vi "Handle.vi"(10 "log record":T1 {"timestamp" format="%<%x %.3X>T"}, 11 "string handler in":refnum<class "String Handler.lvclass">) -> (0 "writer error":errorcluster, 1 "formatter error":errorcluster, 3 "string handler out":refnum<class "String Handler.lvclass">)   [LabVIEW 2024, in "Logging.lvlib" / "String Handler.lvclass"]
uses:
  String Handler.lvclass
  String Handler.lvclass/String Handler.ctl
  Formatters/Formatter/Formatter.lvclass
  Log Record.ctl
  Logging.lvlib
  Logger/Internal Log Levels.ctl
panel:
  # "Connector Pane"
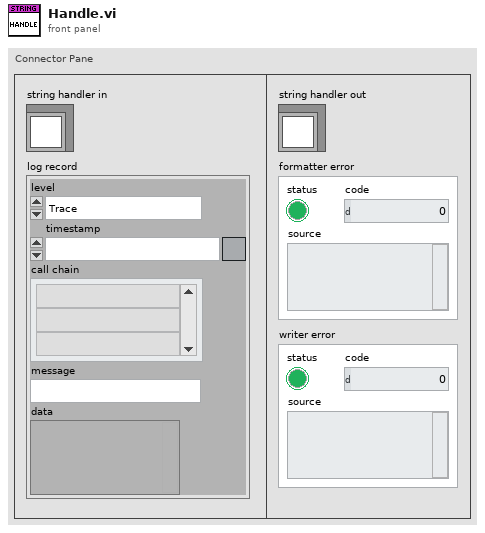
[diagram p1: front panel]
types:
  T1 = typedef "Logging.lvlib/Log Record.ctl" = cluster{"level":T2, "timestamp":timestamp, "call chain":string[], "message":string, "data":variant}
  T2 = typedef "Logging.lvlib/Internal Log Levels.ctl" = enum16{"Trace", "Debug", "Info", "Warning", "Error", "Critical", "Internal"}
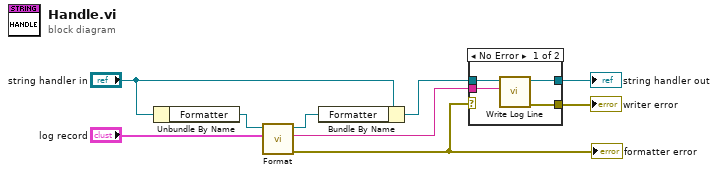
[diagram p0: block diagram]
diagram:
  n1 = Unbundle By Name("string handler in") -> ("Formatter"=w8:refnum<class "Formatter.lvclass">)
  n2 = call-dynamic "Format.vi"("log record"="log record", "formatter in"=w8) -> ("error out"=w2:errorcluster, "log line"=w1:string, "formatter out"=w6:refnum<class "Formatter.lvclass">)  [unwired: 7 in]
  "formatter error" <- w2
  n3 = Bundle By Name(cluster="string handler in", "Formatter"=w6) -> (w5:refnum<class "String Handler.lvclass">)
  n4 = case shown="No Error" w2 {
    tunnel: w5 -> [w13 w14]
    tunnel: [w12 w14] -> w4
    tunnel: [w11 _] -> w3
    tunnel: w1 -> [w10 _]
    frame No Error {
      n5 = call-dynamic "Write Log Line.vi"("log line"=w10, "string handler in"=w13) -> ("error out"=w11:errorcluster, "string handler out"=w12:refnum<class "String Handler.lvclass">)  [unwired: 8 in]
    }
    frame Error {
    }
  }
  "string handler out" <- w4
  "writer error" <- w3
